vi "CurveExport.vi"(8 "error in (no error)":errorcluster caption="entrée d'erreur (pas d'erreur)", 10 "Curves":i32[](array[numeric]), 11 "Interface en entrée":refnum<class "Interface.lvclass"> caption="Interface Class in") -> (0 "error out":errorcluster caption="sortie d'erreur")   [LabVIEW 2019, in "Interface.lvclass"]
uses:
  Interface.lvclass
  CurveSetup.ctl
  Interface.lvclass/Interface.ctl
panel:
  out "Init":bool
  in  "Y Data Name":string
  in  "SepScale":bool caption="Use Separate Scale"
  in  "X Parameter":u16(ring)
  in  "X Data Name":string
  in  "Export":bool
  in  "Y Scale Name":string
  in  "X Scale Name":string
  in  "Courbes":u16(ring)
  in  "stop":bool
  out "Table":string
  in  "Curve Name":string
  out "Current Task":i32=-1
  out "ScanInd":i32
  in  "DisplayName":string
  out "CrvParam":T1[](array[typedef])
  out "NomDon":string[](array[string])=["RTêta;", "X&Y;"]
  out "VarParams":string[](array[string])
  in  "ScanParam":u16(ring) caption="Scan Parameter"
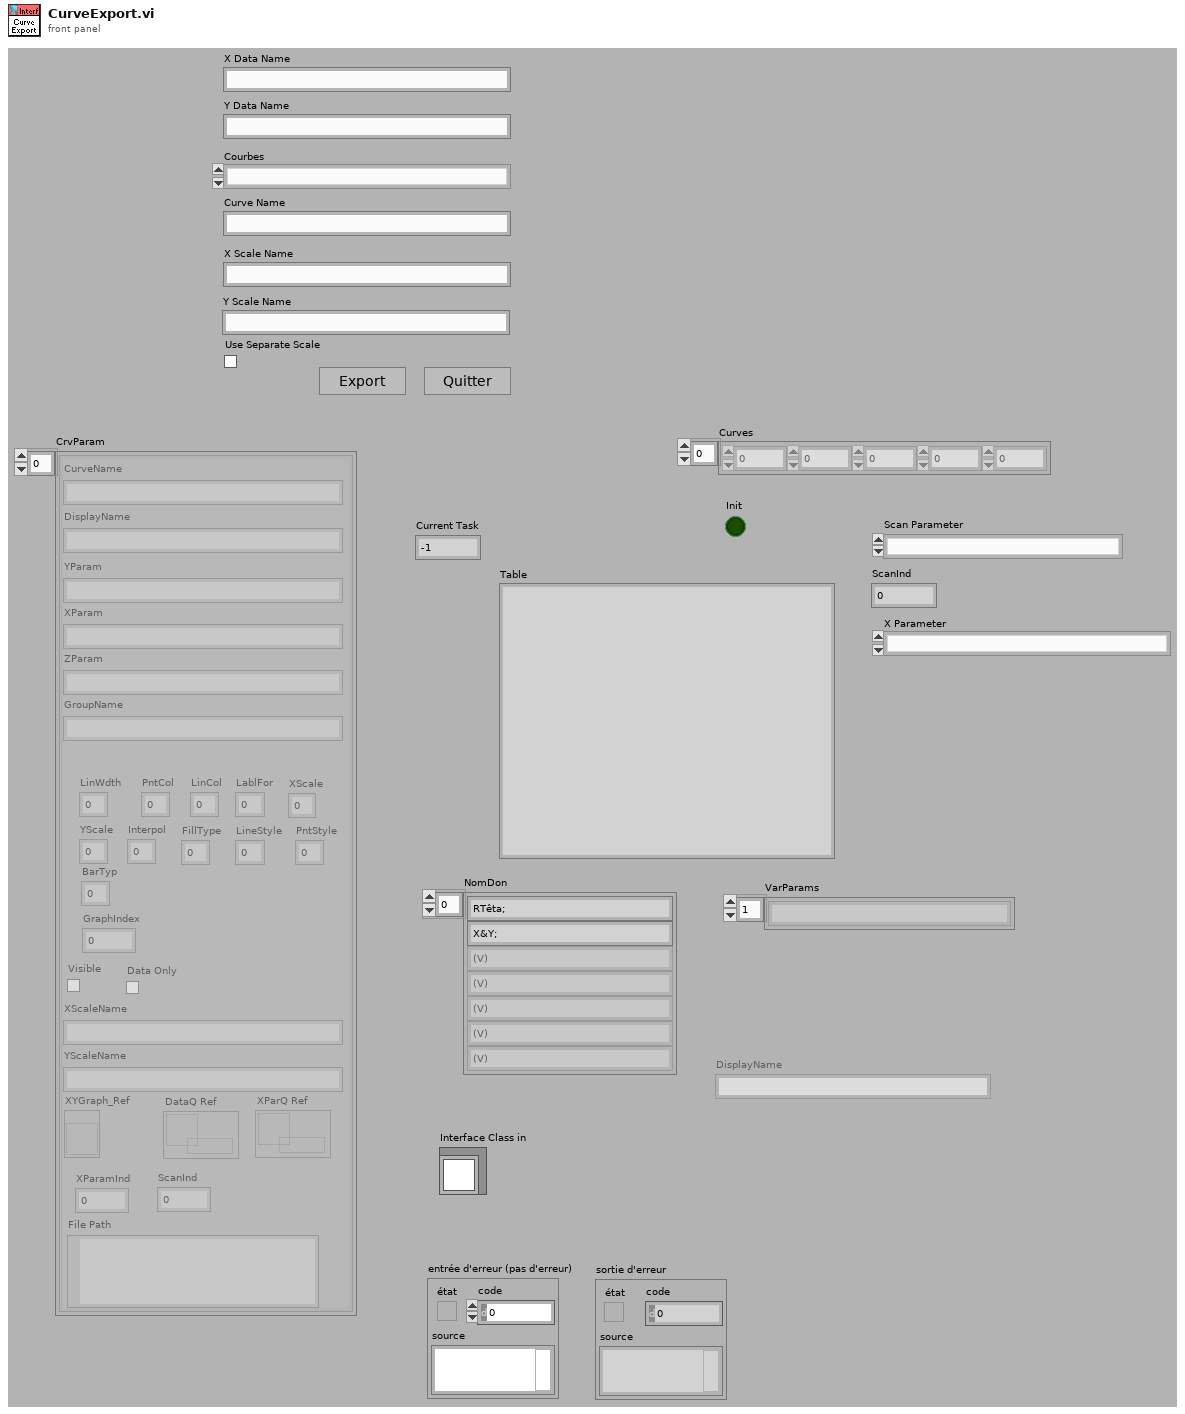
[diagram p1: front panel]
types:
  T1 = typedef "Interface.lvclass/CurveSetup.ctl" = cluster{"CurveName":string, "YParam":string, "XParam":string, "ZParam ":string, "GroupName":string, "LinWdth":u8, "PntCol":u32, "LinCol":u32, "LablFor":u8, "XScale":u32, "YScale":u32, "Interpol":u8, "DisplayName":string, "FillType":i16, "LineStyle":u8, "PntStyle":u8, "BarTyp":u8, "GraphIndex":i32, "Visible":bool, "XScaleName":string, "YScaleName":string, "XYGraph_Ref":refnum<vi>, "Data Only":bool, "DataQ Ref":refnum<queue>, "XParQ Ref":refnum<queue>, "XParamInd":i32, "ScanInd":i32, "File Path":path}
  T2 = enum16{"open", "replace", "create", "open or create", "replace or create", "replace or create with confirmation"}
  T3 = typedef "Interface.lvclass/ScanParams.ctl" = cluster{"Entête":string, "Scan list":string[], "NbCourbe":i32, "IndCourbe":i64, "NomDon":string[], "Session ":i32, "Date":string, "Time":string, "VarParams":string[][], "UserName":string, "ScanTableSize":i32[], "VarPar list":string[], "DescKeyword":string}
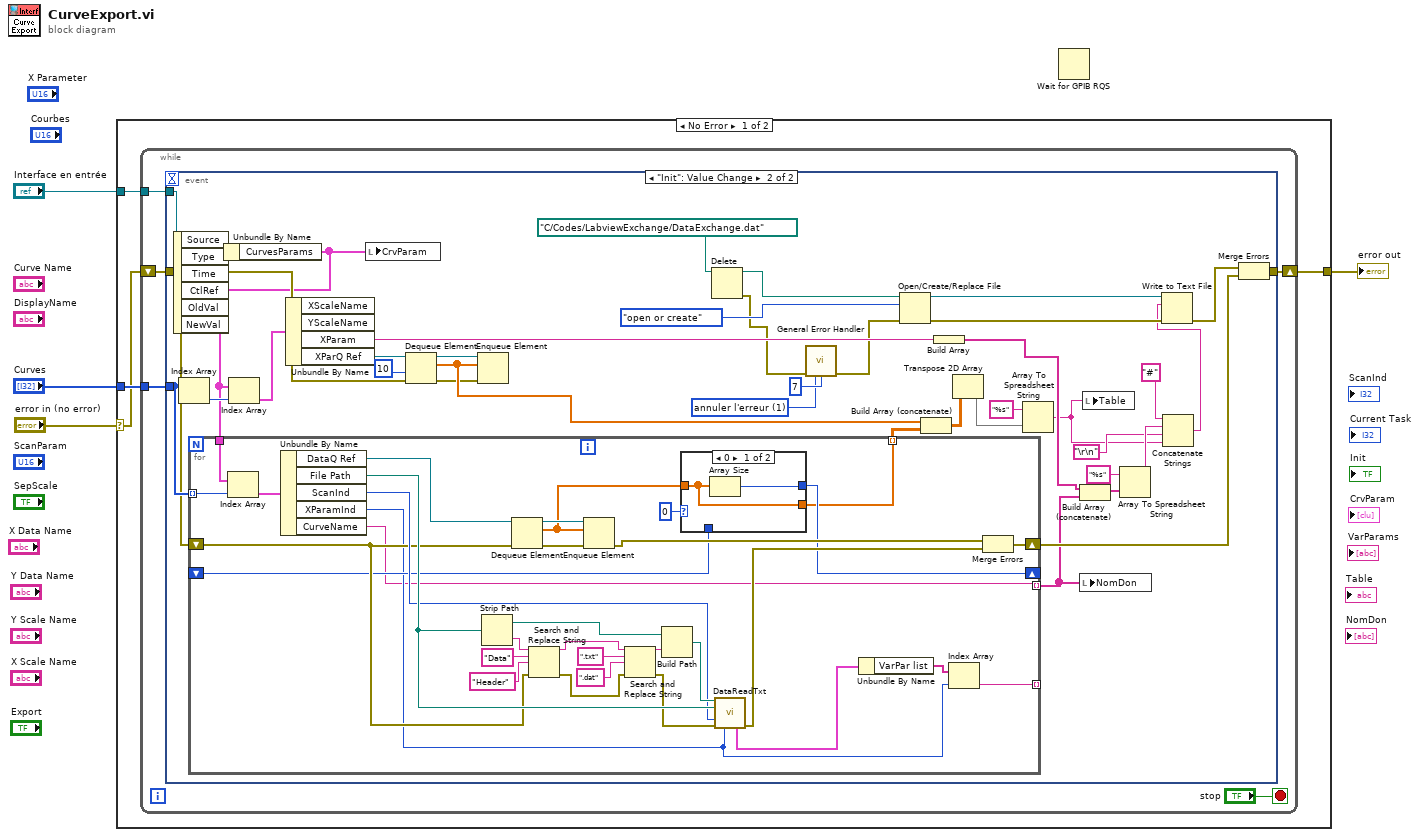
[diagram p0: block diagram]
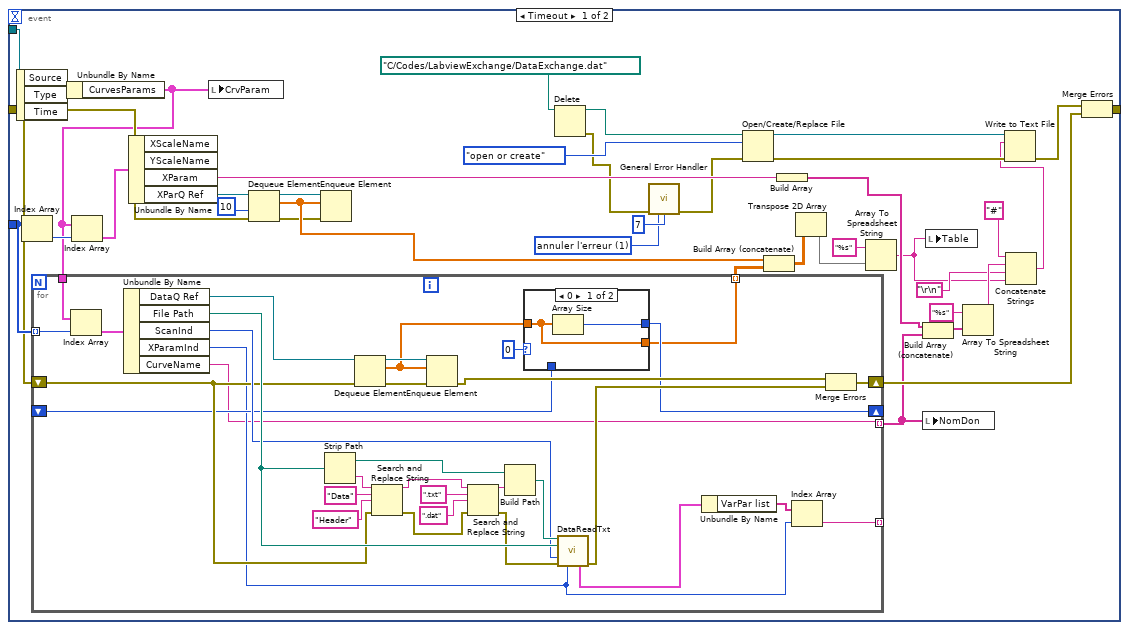
[diagram p2: hidden frame]
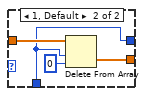
[diagram p3: hidden frame]
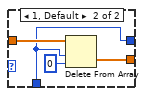
[diagram p4: hidden frame]
diagram:
  n1 = case shown="No Error" "error in (no error)" {
    selector: "error in (no error)" -> [w7 w166]
    tunnel: [w5 w166] -> w3
    tunnel: "Interface en entrée" -> [w6 _]
    tunnel: "Curves" -> [w8 _]
    frame No Error {
      n2 = while {
        tunnel: w8 -> [w13]
        tunnel: w6 -> [w11]
        shift-right: [w10] -> w5
        shift-left: w7 -> [w12]
        stop <- "stop" stop-if-true
        n3 = event shown="[1] \"Init\": Value Change" {
          selector: _ -> [_ _]
          dyn-events: _ -> [_ _]
          timeout: _ -> [_ _]
          tunnel: w13 -> [w43 w119]
          tunnel: w12 -> [w41 w117]
          tunnel: w11 -> [w38 w114]
          tunnel: [w21 w97] -> w10
          event Timeout {
            w18 = 1 items=["pas d'exception", "annuler l'erreur", "définir l'erreur"] ("[exception action] (none:0)")
            n4 = event-data() -> ()  [unwired: 1 in, 3 out]
            n5 = Index Array(array=w43) -> (element=w46:i32)  [unwired: 1 in]
            n6 = Unbundle By Name(w38) -> ("CurvesParams"=w16:T1[])
            n7 = for {
              tunnel: [w56] -> w42 mode=indexing
              tunnel: w16 -> [w65]
              tunnel: w43 -> [w63] mode=indexing
              shift-right: [w60] -> w17
              shift-left: w41 -> [w66]
              shift-right: [w58] -> _
              shift-left: _ -> [w57]
              tunnel: [w52] -> w14 mode=indexing
              tunnel: [w51] -> _ mode=indexing
              n8 = Index Array(array=w65, index=w63) -> (element=w64:T1)
              n9 = Unbundle By Name(w64) -> ("DataQ Ref"=w81:refnum<queue>, "File Path"=w80:path, "ScanInd"=w67:i32, "XParamInd"=w53:i32, "CurveName"=w52:string)
              n10 = Strip Path(path=w80) -> (stripped path=w76:path, name=w79:string)
              n11 = Dequeue Element(queue=w81, error in (no error)=w66) -> (queue out=w82:refnum<queue>, element=w59:dbl[], error out=w83:errorcluster)  [unwired: 1 in, 1 out]
              n12 = Search and Replace String(input string=w79, search string="Data" ("chaîne recherchée"), replace string="Header" ("chaîne de remplacement (\"\")"), error in=w66) -> (result string=w71:string, error out=w73:errorcluster)  [unwired: 4 in, 2 out]
              n13 = Enqueue Element(queue=w82, element=w59, error in (no error)=w83) -> (error out=w61:errorcluster)  [unwired: 1 in, 2 out]
              n14 = Search and Replace String(input string=w71, search string=".txt" ("chaîne recherchée"), replace string=".dat" ("chaîne de remplacement (\"\")"), error in=w73) -> (result string=w69:string, error out=w70:errorcluster)  [unwired: 4 in, 2 out]
              n15 = Build Path(base path=w76, name or relative path=w69) -> (appended path=w75:path)
              n16 = case shown="0" 0 {
                tunnel: w59 -> [w84 w88]
                tunnel: [w85 w86] -> w58
                tunnel: w57 -> [_ w86]
                tunnel: [w84 w87] -> w56
                frame 0 {
                  n17 = Array Size(array=w84) -> (size(s)=w85:i32)
                }
                frame 1, Default {
                  n18 = Delete From Array(array=w88, length=w86, index=0 ("indice")) -> (deleted portion=w87:dbl[])  [unwired: 1 out]
                }
              }
              n19 = call "DataReadTxt.vi"("Chemin Header"=w75, "chemin Data"=w80, "ScanlistIndex"=w67, "error in"=w70, "VarParIndex"=w53) -> ("enregistrement(s)"=w68:T3, "error out"=w62:errorcluster)  [unwired: 3 in, 6 out]
              n20 = Unbundle By Name(w68) -> ("VarPar list"=w54:string[])
              n21 = Index Array(array=w54, index=w53) -> (element=w51:string)
              n22 = Merge Errors(w61, w62) -> (w60:errorcluster)
            }
            n23 = Index Array(array=w16, index=w46) -> (element=w45:T1)
            n24 = Unbundle By Name(w45) -> ("XParam"=w40:string, "XParQ Ref"=w44:refnum<queue>)  [unwired: 2 out]
            n25 = local write "CrvParam"(w16) -> ()
            n26 = Dequeue Element(queue=w44, timeout in ms (-1)=10 ("timeout en ms (-1)"), error in (no error)=w41) -> (queue out=w48:refnum<queue>, element=w49:dbl[], error out=w47:errorcluster)  [unwired: 1 out]
            n27 = Enqueue Element(queue=w48, element=w49, error in (no error)=w47) -> ()  [unwired: 1 in, 3 out]
            n28 = Delete(path (use dialog)=path "C:/Codes/LabviewExchange/DataExchange.dat" ("chemin du fichier (utiliser une boîte de dialogue)")) -> (deleted path=w32:path, error out=w31:errorcluster)  [unwired: 4 in, 1 out]
            n29 = call <vilib>:"General Error Handler.vi"("error in (no error)"=w31, "[exception action] (none:0)"=w18, "[exception code]"=7) -> ("error out"=w20:errorcluster)  [unwired: 8 in, 4 out]
            n30 = Open/Create/Replace File(file path (use dialog)=w32, error in=w20, operation (0:open)=T2."open or create" ("opération (0 : open)")) -> (refnum out=w35:refnum<file>, error out=w30:errorcluster)  [unwired: 3 in, 1 out]
            n31 = Build Array (concatenate)(w49, w42) -> (w37:dbl[][])
            n32 = Build Array(w40) -> (w29:string[])
            n33 = Transpose 2D Array(2D array=w37) -> (transposed array=w36:dbl[][])
            n34 = Array To Spreadsheet String(array=w36, 3:"%s" ("chaîne de format")) -> (spreadsheet string=w15:string)  [unwired: 1 in]
            n35 = Build Array (concatenate)(w29, w14) -> (w27:string[])
            n36 = local write "NomDon"(w14) -> ()
            n37 = local write "Table"(w15) -> ()
            n38 = Array To Spreadsheet String(array=w27, 3:"%s" ("chaîne de format")) -> (spreadsheet string=w26:string)  [unwired: 1 in]
            n39 = Concatenate Strings("#" ("chaîne"), w26, "\r\n", w15) -> (w23:string)
            n40 = Write to Text File(file (use dialog)=w35, text=w23, error in=w30) -> (error out=w22:errorcluster)  [unwired: 1 in, 2 out]
            n41 = Merge Errors(w22, w17) -> (w21:errorcluster)
          }
          event "Init": Value Change {
            w94 = 1 items=["pas d'exception", "annuler l'erreur", "définir l'erreur"] ("[exception action] (none:0)")
            n42 = event-data() -> ()  [unwired: 1 in, 6 out]
            n43 = Index Array(array=w119) -> (element=w122:i32)  [unwired: 1 in]
            n44 = Unbundle By Name(w114) -> ("CurvesParams"=w92:T1[])
            n45 = for {
              tunnel: [w132] -> w118 mode=indexing
              tunnel: w92 -> [w141]
              tunnel: w119 -> [w139] mode=indexing
              shift-right: [w136] -> w93
              shift-left: w117 -> [w142]
              shift-right: [w134] -> _
              shift-left: _ -> [w133]
              tunnel: [w128] -> w90 mode=indexing
              tunnel: [w127] -> _ mode=indexing
              n46 = Index Array(array=w141, index=w139) -> (element=w140:T1)
              n47 = Unbundle By Name(w140) -> ("DataQ Ref"=w157:refnum<queue>, "File Path"=w156:path, "ScanInd"=w143:i32, "XParamInd"=w129:i32, "CurveName"=w128:string)
              n48 = Strip Path(path=w156) -> (stripped path=w152:path, name=w155:string)
              n49 = Dequeue Element(queue=w157, error in (no error)=w142) -> (queue out=w158:refnum<queue>, element=w135:dbl[], error out=w159:errorcluster)  [unwired: 1 in, 1 out]
              n50 = Search and Replace String(input string=w155, search string="Data" ("chaîne recherchée"), replace string="Header" ("chaîne de remplacement (\"\")"), error in=w142) -> (result string=w147:string, error out=w149:errorcluster)  [unwired: 4 in, 2 out]
              n51 = Enqueue Element(queue=w158, element=w135, error in (no error)=w159) -> (error out=w137:errorcluster)  [unwired: 1 in, 2 out]
              n52 = Search and Replace String(input string=w147, search string=".txt" ("chaîne recherchée"), replace string=".dat" ("chaîne de remplacement (\"\")"), error in=w149) -> (result string=w145:string, error out=w146:errorcluster)  [unwired: 4 in, 2 out]
              n53 = Build Path(base path=w152, name or relative path=w145) -> (appended path=w151:path)
              n54 = case shown="0" 0 {
                tunnel: w135 -> [w160 w164]
                tunnel: [w161 w162] -> w134
                tunnel: w133 -> [_ w162]
                tunnel: [w160 w163] -> w132
                frame 0 {
                  n55 = Array Size(array=w160) -> (size(s)=w161:i32)
                }
                frame 1, Default {
                  n56 = Delete From Array(array=w164, length=w162, index=0 ("indice")) -> (deleted portion=w163:dbl[])  [unwired: 1 out]
                }
              }
              n57 = call "DataReadTxt.vi"("Chemin Header"=w151, "chemin Data"=w156, "ScanlistIndex"=w143, "error in"=w146, "VarParIndex"=w129) -> ("enregistrement(s)"=w144:T3, "error out"=w138:errorcluster)  [unwired: 3 in, 6 out]
              n58 = Unbundle By Name(w144) -> ("VarPar list"=w130:string[])
              n59 = Index Array(array=w130, index=w129) -> (element=w127:string)
              n60 = Merge Errors(w137, w138) -> (w136:errorcluster)
            }
            n61 = Index Array(array=w92, index=w122) -> (element=w121:T1)
            n62 = Unbundle By Name(w121) -> ("XParam"=w116:string, "XParQ Ref"=w120:refnum<queue>)  [unwired: 2 out]
            n63 = local write "CrvParam"(w92) -> ()
            n64 = Dequeue Element(queue=w120, timeout in ms (-1)=10 ("timeout en ms (-1)"), error in (no error)=w117) -> (queue out=w124:refnum<queue>, element=w125:dbl[], error out=w123:errorcluster)  [unwired: 1 out]
            n65 = Enqueue Element(queue=w124, element=w125, error in (no error)=w123) -> ()  [unwired: 1 in, 3 out]
            n66 = Delete(path (use dialog)=path "C:/Codes/LabviewExchange/DataExchange.dat" ("chemin du fichier (utiliser une boîte de dialogue)")) -> (deleted path=w108:path, error out=w107:errorcluster)  [unwired: 4 in, 1 out]
            n67 = call <vilib>:"General Error Handler.vi"("error in (no error)"=w107, "[exception action] (none:0)"=w94, "[exception code]"=7) -> ("error out"=w96:errorcluster)  [unwired: 8 in, 4 out]
            n68 = Open/Create/Replace File(file path (use dialog)=w108, error in=w96, operation (0:open)=T2."open or create" ("opération (0 : open)")) -> (refnum out=w111:refnum<file>, error out=w106:errorcluster)  [unwired: 3 in, 1 out]
            n69 = Build Array (concatenate)(w125, w118) -> (w113:dbl[][])
            n70 = Build Array(w116) -> (w105:string[])
            n71 = Transpose 2D Array(2D array=w113) -> (transposed array=w112:dbl[][])
            n72 = Array To Spreadsheet String(array=w112, 3:"%s" ("chaîne de format")) -> (spreadsheet string=w91:string)  [unwired: 1 in]
            n73 = Build Array (concatenate)(w105, w90) -> (w103:string[])
            n74 = local write "NomDon"(w90) -> ()
            n75 = local write "Table"(w91) -> ()
            n76 = Array To Spreadsheet String(array=w103, 3:"%s" ("chaîne de format")) -> (spreadsheet string=w102:string)  [unwired: 1 in]
            n77 = Concatenate Strings("#" ("chaîne"), w102, "\r\n", w91) -> (w99:string)
            n78 = Write to Text File(file (use dialog)=w111, text=w99, error in=w106) -> (error out=w98:errorcluster)  [unwired: 1 in, 2 out]
            n79 = Merge Errors(w98, w93) -> (w97:errorcluster)
          }
        }
      }
    }
    frame Error {
    }
  }
  "error out" <- w3
  n80 = Wait for GPIB RQS() -> ()  [unwired: 3 in, 2 out]
